vi "Vision Research Phantom Series PhCon PhGetCameraOptions.vi"(0 "CN in":u32=1, 5 "Error In (no error)":errorcluster) -> (14 "CN out":u32=1, 16 "CAMERAOPTIONS":T1 {"VideoSystem" items=["VIDEOSYS_NTSC"=0, "VIDEOSYS_PAL"=1, "VIDEOSYS_720P60"=4, "VIDEOSYS_720P59DOT9"=12, "VIDEOSYS_720P50"=5, "VIDEOSYS_1080P30"=20, "VIDEOSYS_1080P29DOT9"=28, "VIDEOSYS_1080P25"=21, "VIDEOSYS_1080P24"=36, "VIDEOSYS_1080P23DOT9"=44, "VIDEOSYS_1080I30"=68, "VIDEOSYS_1080I29DOT9"=76, "VIDEOSYS_1080I25"=69, "VIDEOSYS_1080PSF30"=52, "VIDEOSYS_1080PSF29DOT9"=60, "VIDEOSYS_1080PSF25"=53, "VIDEOSYS_1080PSF24"=84, "VIDEOSYS_1080PSF23DOT9"=92]}, 19 "Error Out":errorcluster)   [LabVIEW 2013, in "VRI.lvlib"]
doc: "PhCon dll\n\nPhGetCameraOptions\nHRESULT PhGetCameraOptions(UINT CN, PCAMERAOPTIONS pOptions);\n\nParameters Description\nCN (in) Camera number\npOptions (out) Pointer to the camera options\nReturn HRESULT (0=Ok)\nComments Transfer the current settings of the general options to the caller.\n\n\nWritten by:\nBLOOMY CONTROLS, INC\nWINDSOR, CT 06095, USA\n860-298-9925\nwww.bloomy.com\nV1.0.0\nMay, 2004"
uses:
  VRI.lvlib
  _Type Defs/PHCon CAMERAOPTIONS.ctl
  _Type Defs/PhCon VideoSystem.ctl
  _Type Defs/RGBQUAD.ctl
  _Type Defs/PHCon IMRANGE.ctl
  Phantom DLLs/PhCon.dll
panel:
  out "CamOpt Data":u32[](array[numeric])
  # "For instructions on the use of this VI, press Ctrl+H to display the help window and move the mouse over the icon, controls, and indicators"
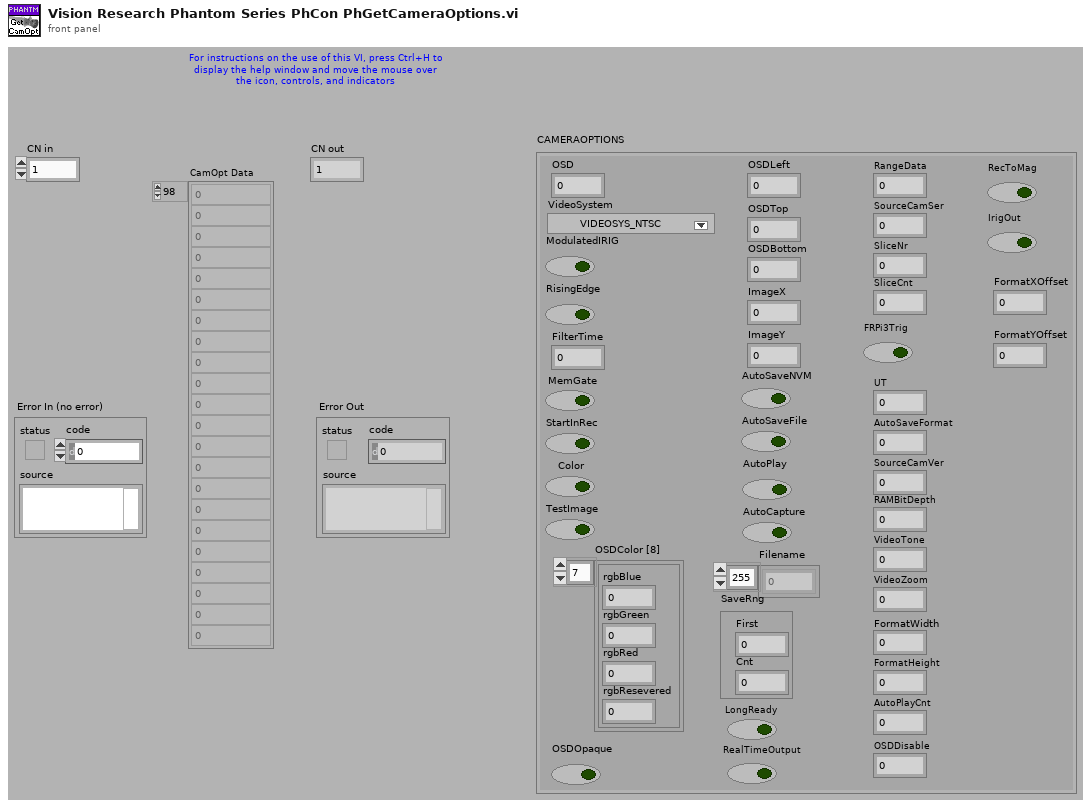
[diagram p1: front panel]
types:
  T1 = typedef "VRI.lvlib/PHCon CAMERAOPTIONS.ctl" = cluster{"OSD":u32, "VideoSystem":T2, "ModulatedIRIG":bool, "RisingEdge":bool, "FilterTime":u32, "MemGate":bool, "StartInRec":bool, "Color":bool, "TestImage":bool, "OSDColor [8]":T3[], "OSDOpaque":bool, "OSDLeft":i32, "OSDTop":i32, "OSDBottom":i32, "ImageX":i32, "ImageY":i32, "AutoSaveNVM":bool, "AutoSaveFile":bool, "AutoPlay":bool, "AutoCapture":bool, "Filename":u8[], "SaveRng":T4, "LongReady":bool, "RealTimeOutput":bool, "RangeData":u32, "SourceCamSer":u32, "SliceNr":u32, "SliceCnt":u32, "FRPi3Trig":bool, "UT":u32, "AutoSaveFormat":i8, "SourceCamVer":u32, "RAMBitDepth":u32, "VideoTone":i32, "VideoZoom":i32, "FormatWidth":i32, "FormatHeight":i32, "AutoPlayCnt":u32, "OSDDisable":u32, "RecToMag":bool, "IrigOut":bool, "FormatXOffset":i32, "FormatYOffset":i32}
  T2 = typedef "VRI.lvlib/PhCon VideoSystem.ctl" = u32
  T3 = typedef "VRI.lvlib/RGBQUAD.ctl" = cluster{"rgbBlue":u8, "rgbGreen":u8, "rgbRed":u8, "rgbResevered":u8}
  T4 = typedef "VRI.lvlib/PHCon IMRANGE.ctl" = cluster{"First":i32, "Cnt":u32}
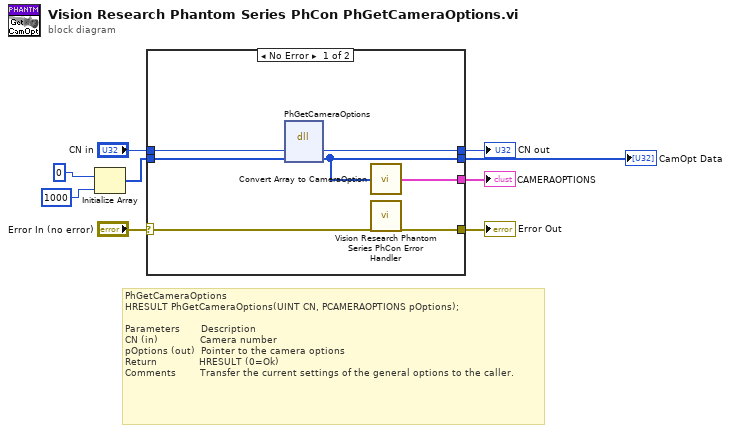
[diagram p0: block diagram]
diagram:
  # "PhGetCameraOptions\nHRESULT PhGetCameraOptions(UINT CN, PCAMERAOPTIONS pOptions);\n\nParameters       Description\nCN (in)              Camera number\npOptions (out)  Pointer to the camera options\nReturn              HRESULT (0=Ok)\nComments        Transfer the current settings of the general options to the caller."
  n1 = Initialize Array(u32 0, 1000) -> (w1:u32[])
  n2 = case shown="No Error" "Error In (no error)" {
    selector: "Error In (no error)" -> [w16 w19]
    tunnel: [w15 w19] -> w8
    tunnel: "CN in" -> [w14 w18]
    tunnel: [w13 w18] -> w6
    tunnel: w1 -> [w12 w17]
    tunnel: [w11 w17] -> w5
    tunnel: [w10 _] -> w4
    frame No Error {
      n3 = dll-call lib="C:/Projects/SDK/32-bit/Vision Research Phantom Series Labview Driver/Phantom DLLs/PhCon.dll" fn="PhGetCameraOptions"("CN"=w14, "pOptions"=w12) -> ("CN"=w13:u32, "pOptions"=w11:u32[])  [unwired: 3 in, 3 out]
      n4 = call "Convert Array to CameraOption.vi"("CAMERAOPTIONS Data"=w11) -> ("CAMERAOPTIONS"=w10:T1)
      n5 = call "Vision Research Phantom Series PhCon Error Handler.vi"("Error In (no error)"=w16) -> ("Error Out"=w15:errorcluster)  [unwired: 1 in, 17 out]
    }
    frame Error {
    }
  }
  "Error Out" <- w8
  "CN out" <- w6
  "CamOpt Data" <- w5
  "CAMERAOPTIONS" <- w4
